vi "Read Speed.vi"(8 "error in":errorcluster, 10 "Speeds Label":string, 11 "Config Files Path":path) -> (0 "error out":errorcluster, 2 "Speed":dbl)   [LabVIEW 2011]
uses:
  <vilib>/Utility/config.llb/Read Key (Double).vi
  <vilib>/Utility/config.llb/NI_LVConfig.lvlib
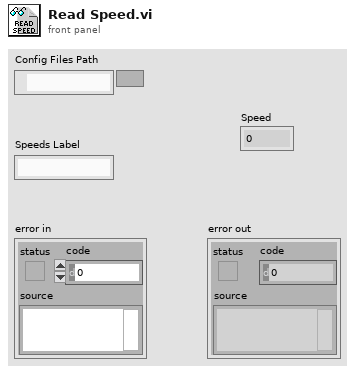
[diagram p1: front panel]
types:
  T1 = typedef "NI_LVConfig.lvlib/Config Data RefNum.ctl" = refnum<k1>
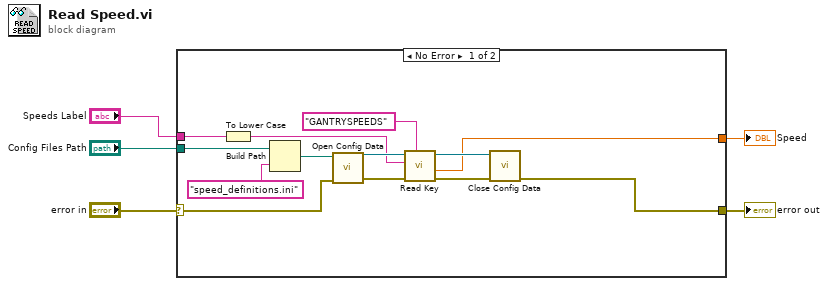
[diagram p0: block diagram]
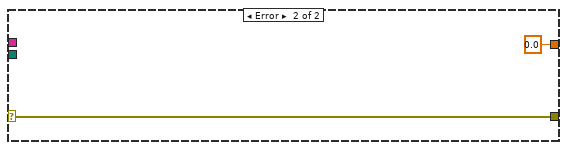
[diagram p2: hidden frame]
diagram:
  n1 = case shown="No Error" "error in" {
    selector: "error in" -> [w15 w20]
    tunnel: [w7 w20] -> w4
    tunnel: "Config Files Path" -> [w18 _]
    tunnel: "Speeds Label" -> [w12 _]
    tunnel: [w6 0.0 ("value")] -> w1
    frame No Error {
      n2 = To Lower Case(string=w12) -> (all lower case string=w11:string)
      n3 = Build Path(base path=w18, name or relative path="speed_definitions.ini") -> (appended path=w16:path)
      n4 = call <vilib>:"Open Config Data.vi"("error in (no error)"=w15, "configuration file path"=w16) -> ("error out"=w10:errorcluster, "refnum"=w14:T1)  [unwired: 7 in, 1 out]
      n5 = call-poly <vilib>:"Read Key.vi"("section"="GANTRYSPEEDS", "error in (no error)"=w10, "key"=w11, "refnum"=w14) -> ("error out"=w8:errorcluster, "value"=w6:dbl, "refnum out"=w9:T1)  [unwired: 4 in, 1 out]
      n6 = call <vilib>:"Close Config Data.vi"("error in (no error)"=w8, "refnum"=w9) -> ("error out"=w7:errorcluster)  [unwired: 8 in, 1 out]
    }
    frame Error {
    }
  }
  "error out" <- w4
  "Speed" <- w1
